vi "Read channels.vi"(8 "error in (no error)":errorcluster, 11 "Conditional Jump Step Config in":refnum<class "Conditional Jump Step Config.lvclass">) -> (0 "error out":errorcluster, 2 "Channels":refnum<class "TBM channel.lvclass">[](array[class]), 3 "Conditional Jump Step Config out":refnum<class "Conditional Jump Step Config.lvclass">)   [LabVIEW 2015, in "Conditional Jump Step Config.lvclass"]
uses:
  Conditional Jump Step Config.lvclass
  <vilib>/NI/Tag Bus Module Framework/channel/TBM channel.lvclass
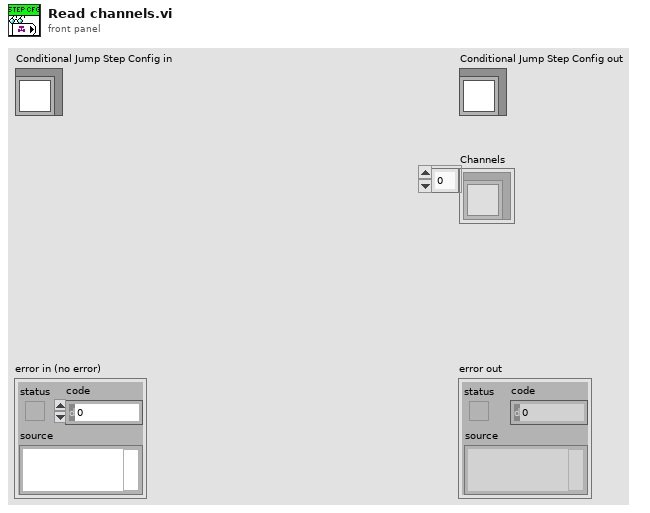
[diagram p1: front panel]
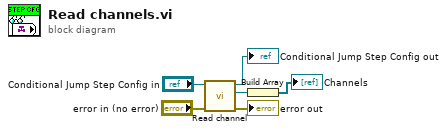
[diagram p0: block diagram]
diagram:
  n1 = call-dynamic "Read channel.vi"("error in (no error)"="error in (no error)", "Conditional Jump Step Config in"="Conditional Jump Step Config in") -> ("error out"=→"error out":errorcluster, "channel"=w2:refnum<class "TBM channel.lvclass">, "Conditional Jump Step Config out"=→"Conditional Jump Step Config out":refnum<class "Conditional Jump Step Config.lvclass">)  [unwired: 7 in]
  n2 = Build Array(w2) -> (→"Channels":refnum<class "TBM channel.lvclass">[])
